vi "Cmd_U16U32.vi"(5 "Arg2":u32 max=127 step=1, 7 "Arg1":u16 max=127 step=1, 8 "error in (no error)":errorcluster, 9 "Cmd":u8, 10 "Address":u8, 11 "VISA Refnum in":refnum<visa-resource-name>) -> (0 "error out":errorcluster, 2 "Valid":bool, 3 "VISA Refnum out":refnum<visa-resource-name>)   [LabVIEW 2015, in "Ion Motion Roboclaw.lvlib"]
uses:
  <instrlib>/Ion Motion Roboclaw/Ion Motion Roboclaw.lvlib
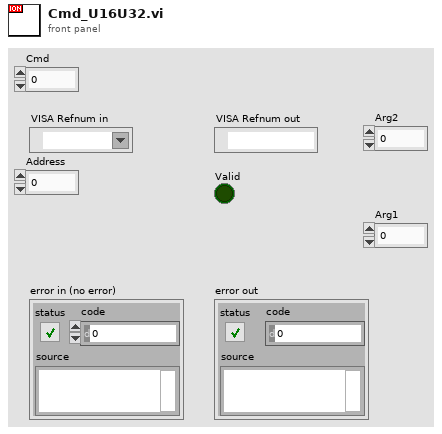
[diagram p1: front panel]
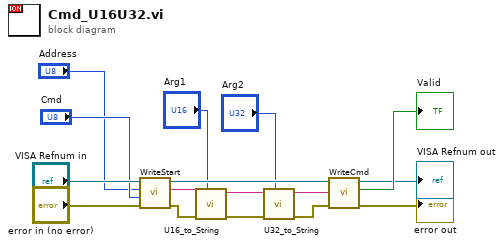
[diagram p0: block diagram]
diagram:
  n1 = call <instrlib>:"WriteStart.vi"("error in (no error)"="error in (no error)", "Cmd"="Cmd", "Address"="Address", "VISA Refnum in"="VISA Refnum in") -> ("error out"=w6:errorcluster, "String Out"=w7:string, "VISA Refnum out"=w9:refnum<visa-resource-name>)  [unwired: 5 in]
  n2 = call <instrlib>:"U16_to_String.vi"("number"="Arg1", "error in (no error)"=w6, "String In"=w7) -> ("error out"=w5:errorcluster, "String Out"=w4:string)  [unwired: 5 in]
  n3 = call <instrlib>:"U32_to_String.vi"("number"="Arg2", "error in (no error)"=w5, "String In"=w4) -> ("error out"=w11:errorcluster, "String Out"=w10:string)  [unwired: 5 in]
  n4 = call <instrlib>:"WriteCmd.vi"("error in (no error)"=w11, "write buffer"=w10, "VISA Refnum in"=w9) -> ("error out"=→"error out":errorcluster, "Valid"=→"Valid":bool, "VISA Refnum out"=→"VISA Refnum out":refnum<visa-resource-name>)  [unwired: 2 in]
